vi "HW_Get_raw_data_flow_from_serial_port.vi"(6 "error in":errorcluster, 8 "VISA resource name in":refnum<visa-resource-name>) -> (0 "Not empty?":bool, 1 "error out":errorcluster, 2 "Timestamp":timestamp, 3 "Data":string, 5 "VISA resource name out":refnum<visa-resource-name>)   [LabVIEW 2018, in "Tracker.lvlib"]
uses:
  Tracker.lvlib
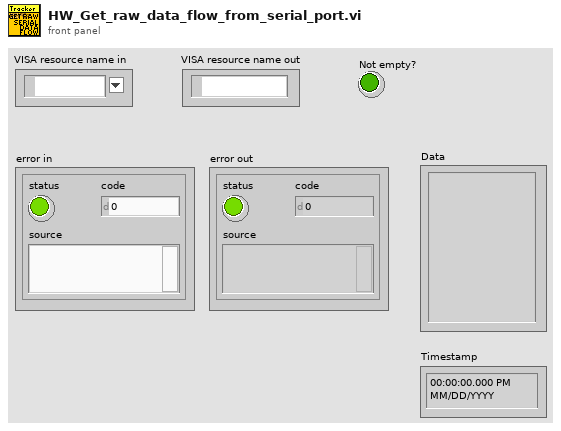
[diagram p1: front panel]
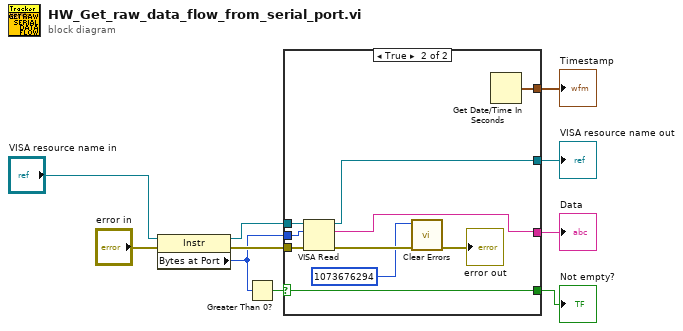
[diagram p0: block diagram]
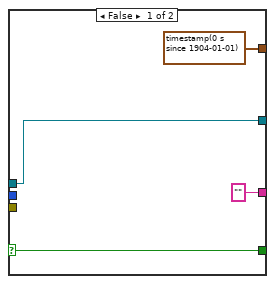
[diagram p2: hidden frame]
diagram:
  n1 = property class="Instr"(reference="VISA resource name in", error in="error in") -> (reference out=w8:refnum<visa-resource-name>, error out=w9:errorcluster, "Bytes at Port"=w7:u32)
  n2 = Greater Than 0?(x=w7) -> (x > 0?=w6:bool)
  n3 = case shown="True" w6 {
    selector: w6 -> [w13 w17]
    tunnel: [w14 w23] -> w4
    tunnel: w7 -> [_ w22]
    tunnel: w9 -> [_ w21]
    tunnel: w8 -> [w14 w20]
    tunnel: [w13 w17] -> w3
    tunnel: ["" w15] -> w2
    tunnel: [timestamp(0 s since 1904-01-01) ("seconds since 1Jan1904") w16] -> w1
    frame False {
    }
    frame True {
      n4 = VISA Read(VISA resource name=w20, byte count=w22, error in (no error)=w21) -> (VISA resource name out=w23:refnum<visa-resource-name>, read buffer=w15:string, error out=w24:errorcluster)  [unwired: 1 out]
      n5 = call <vilib>:"Clear Errors.vi"("error in (no error)"=w24, "specific error code to clear (0: all)"=1073676294) -> ("error out"=→"error out":errorcluster)  [unwired: 4 in, 1 out]
      n6 = Get Date/Time In Seconds ("Current time")() -> (seconds since 1Jan1904=w16:timestamp)
    }
  }
  "VISA resource name out" <- w4
  "Not empty?" <- w3
  "Data" <- w2
  "Timestamp" <- w1
